vi "Get Rich to Flat Info.vi"(10 "oneof container name":string, 11 "field name":string) -> (1 "bundler terminal name":string, 2 "getter vi name":string, 3 "get value terminal name":string)   [LabVIEW 2019, in "gRPC Template Creation Utility.lvlib"]
uses:
  gRPC Template Creation Utility.lvlib
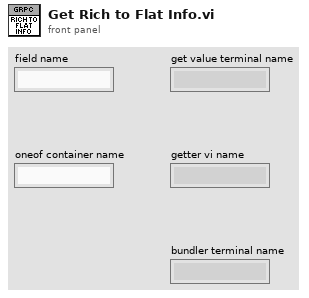
[diagram p1: front panel]
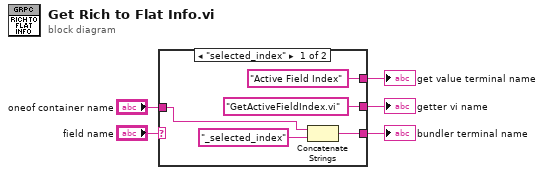
[diagram p0: block diagram]
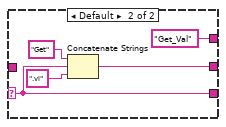
[diagram p2: hidden frame]
diagram:
  n1 = case shown="\"selected_index\"" "field name" {
    selector: "field name" -> [_ w11]
    tunnel: ["GetActiveFieldIndex.vi" w15] -> w1
    tunnel: ["Active Field Index" ("Terminal name") "Get_Val" ("Terminal name")] -> w3
    tunnel: [w6 w11] -> w4
    tunnel: "oneof container name" -> [w8 _]
    frame "selected_index" {
      n2 = Concatenate Strings(w8, "_selected_index" ("string")) -> (w6:string)
    }
    frame Default {
      n3 = Concatenate Strings("Get" ("string"), w11, ".vi" ("string")) -> (w15:string)
    }
  }
  "bundler terminal name" <- w4
  "get value terminal name" <- w3
  "getter vi name" <- w1
